vi "Create Satellite Module LVLib.vi"(6 "Kernel LVLib Path":path=path "C:/LQWidgets/LQ Widgets Core/LQ Widgets Core.lvlib", 7 "Template LVLib Path":path=path "D:/Development/Projects/LQWidgets-CodeGen/templates/LabVIEW/Template.lvlib", 9 "Kernel Module Spec. File":path=path "D:/Development/Projects/LQWidgets-CodeGen/data/LQ Widgets Core.json", 10 "Output Dir":path=path "C:/LQWidgets", 11 "Module Spec. File":path=path "D:/Development/Projects/LQWidgets-CodeGen/data/Qt SVG.json") -> (2 "Module LVLib Path":path)   [LabVIEW 2013]
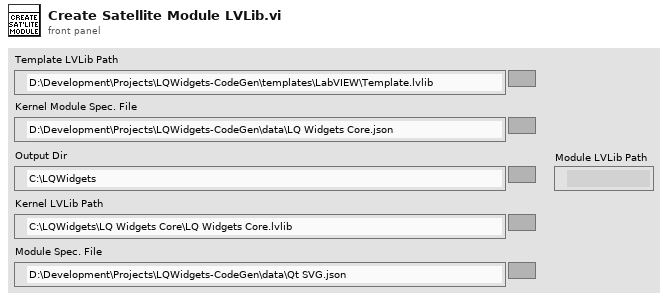
[diagram p1: front panel]
types:
  T1 = typedef "Type Categories.ctl" = cluster{"numerics":T2[], "simpleStructs":T3[], "opaqueStructs":T6[], "simpleIdentities":T6[], "qObjects":T6[], "simpleContainers":T2[], "fullArrays":T2[]}
  T2 = typedef "TypeConv.ctl" = cluster{"name":string, "dllType":string}
  T3 = typedef "Simple Struct.ctl" = cluster{"name":string, "fields":T4[], "methods":T5[]}
  T4 = typedef "Param.ctl" = cluster{"name":string, "type":string}
  T5 = typedef "Method.ctl" = cluster{"name":string, "retType":string, "params":T4[], "isConst":bool, "isStaticMember":bool, "isFactory":bool}
  T6 = typedef "Class.ctl" = cluster{"name":string, "base":string, "enums":T7[], "methods":T5[], "properties":T9[]}
  T7 = typedef "Enum.ctl" = cluster{"name":string, "values":T8[]}
  T8 = typedef "Enum Value.ctl" = cluster{"name":string, "value":i32}
  T9 = typedef "Property.ctl" = cluster{"name":string, "getter":string, "setter":string}
  T10 = typedef "Projection Info.ctl" = cluster{"source":string, "projection":string}
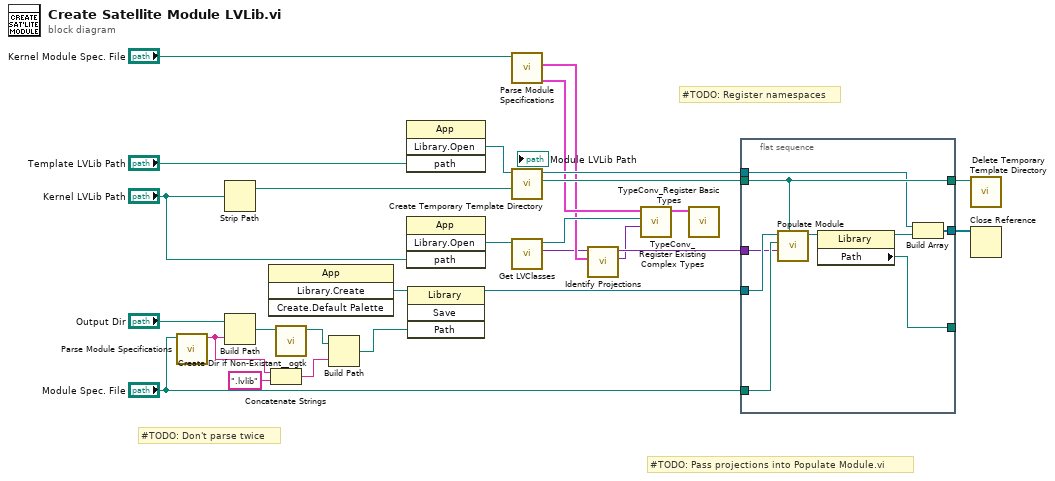
[diagram p0: block diagram]
diagram:
  # "#TODO: Register namespaces"
  # "#TODO: Pass projections into Populate Module.vi"
  # "#TODO: Don't parse twice"
  n1 = call "Parse Module Specifications.vi"("Module Spec. File"="Module Spec. File") -> ("Module Name"=w10:string)  [unwired: 7 in, 3 out]
  n2 = Strip Path(path="Kernel LVLib Path") -> (stripped path=w17:path)  [unwired: 1 out]
  n3 = Build Path(base path="Output Dir", name or relative path=w10) -> (appended path=w14:path)
  n4 = invoke class="App" method="Library.Create"() -> ("Create Library"=w21:refnum<vi>)  [unwired: 4 in, 3 out]
  n5 = Concatenate Strings(w10, ".lvlib" ("string")) -> (w9:string)
  n6 = call <userlib>:"Create Dir if Non-Existant__ogtk.vi"("Directory Path"=w14) -> ("dup Directory Path"=w13:path)  [unwired: 8 in, 2 out]
  n7 = Build Path(base path=w13, name or relative path=w9) -> (appended path=w12:path)
  n8 = invoke class="App" method="Library.Open"("path"="Template LVLib Path") -> ("Open Library"=w22:refnum<vi>)  [unwired: 3 in, 3 out]
  n9 = invoke class="App" method="Library.Open"("path"="Kernel LVLib Path") -> ("Open Library"=w15:refnum<vi>)  [unwired: 3 in, 3 out]
  n10 = invoke class="Library" method="Save"(reference=w21, "Path"=w12) -> (reference out=w20:refnum<vi>)  [unwired: 2 in, 3 out]
  n11 = call "Parse Module Specifications.vi"("Module Spec. File"="Kernel Module Spec. File") -> ("Type Categories"=w6:T1, "Projections"=w5:T10[])  [unwired: 7 in, 2 out]
  n12 = call "Create Temporary Template Directory.vi"("Kernel LVLib Dir"=w17, "Template LVLib"=w22) -> ("Temporary Template Root Dir"=w27:path, "Template LVLib Dup"=w24:refnum<vi>)  [unwired: 8 in]
  n13 = call "Get LVClasses.vi"("LVLib"=w15) -> ("Class Ref Map"=w4:variant, "LVLib Dup"=w8:refnum<vi>)  [unwired: 9 in]
  n14 = call "Identify Projections.vi"("Projection Info"=w5, "Class Ref Map"=w4) -> ("Projection Ref Map"=w2:variant, "Class Ref Map Dup"=w3:variant)  [unwired: 8 in]
  n15 = call "TypeConv_Register Existing Complex Types.vi"("Projection Ref Map"=w2, "Existing Module"=w8, "Type Categories"=w6) -> ("Type Categories Dup"=w1:T1)  [unwired: 8 in]
  n16 = call "TypeConv_Register Basic Types.vi"("Type Categories"=w1) -> ()  [unwired: 10 in, 1 out]
  n17 = flat-sequence {
    tunnel: w27 -> [w34]
    tunnel: w20 -> [w36]
    tunnel: [w32] -> w26
    tunnel: "Module Spec. File" -> [w35]
    tunnel: [w34] -> w25
    tunnel: w24 -> [w33]
    tunnel: w3 -> [w31]
    tunnel: [w28] -> _
    frame #0 {
      n18 = call "Populate Module.vi"("Temporary Template Root Dir"=w34, "Existing LVClass Ref Map"=w31, "Module Spec. File"=w35, "Module LVLib"=w36) -> ("Modified Module LVLib"=w30:refnum<vi>)  [unwired: 7 in]
      n19 = property class="Library"(reference=w30) -> (reference out=w29:refnum<vi>, "Path"=w28:path)  [unwired: 1 in, 1 out]
      n20 = Build Array(w33, w29) -> (w32:refnum<vi>[])
    }
  }
  n21 = call "Delete Temporary Template Directory.vi"("Target Template Root Dir"=w25) -> ()  [unwired: 11 in]
  n22 = Close Reference(reference=w26) -> ()  [unwired: 1 in, 1 out]
